vi "goto_mem_pos.vi"(6 "Speed (um/s)":i32, 8 "error in (no error)":errorcluster, 9 "storage_id":i32, 10 "device ID":i32, 11 "Handle in":i64) -> (0 "error out":errorcluster, 2 "Return (<0 is error)":i32, 3 "Handle out":i64)   [LabVIEW 2016, in "OSB_uMp_library.lvlib"]
doc: "Sends uMp to a previously stored position"
uses:
  OSB_uMp_library.lvlib
  ump.dll
panel:
  # "By Stuart Box at OxSyBio Ltd, 2017\n\nThis software is provided WITHOUT ANY WARRANTY; without even the implied warranty of MERCHANTABILITY or FITNESS FOR A PARTICULAR PURPOSE.\n\ninfo@oxsybio.com\n\nOxSyBio Ltd, The Walbrook Building, 25 Walbrook, London, EC4N 8AF"
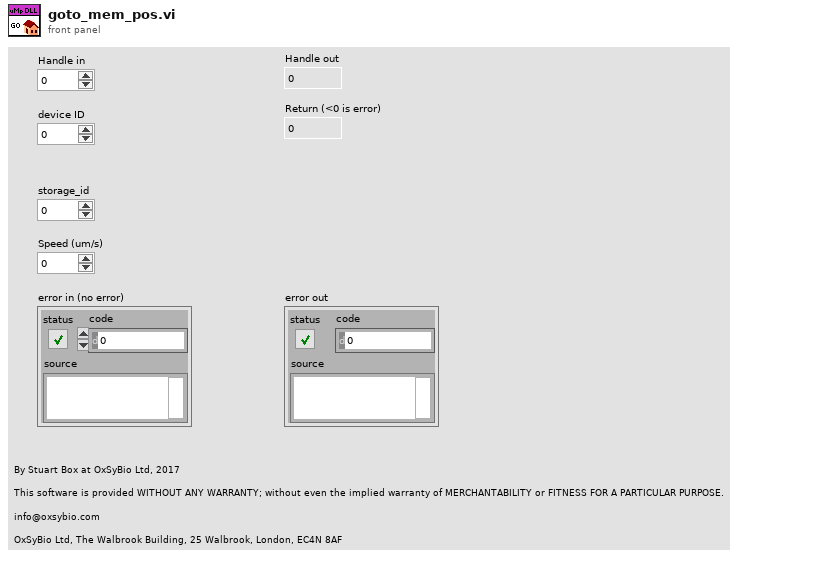
[diagram p1: front panel]
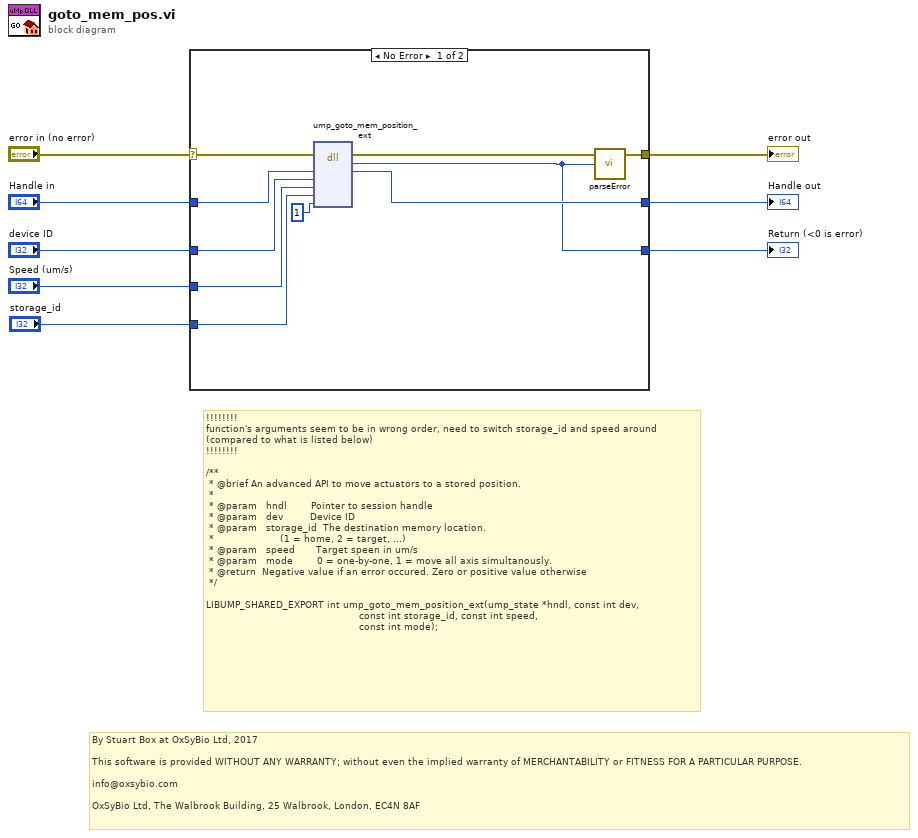
[diagram p0: block diagram]
diagram:
  # "By Stuart Box at OxSyBio Ltd, 2017\n\nThis software is provided WITHOUT ANY WARRANTY; without even the implied warranty of MERCHANTABILITY or FITNESS FOR A PARTICULAR PURPOSE.\n\ninfo@oxsybio.com\n\nOxSyBio Ltd, The Walbrook Building, 25 Walbrook, London, EC4N 8AF"
  # "!!!!!!!!\nfunction's arguments seem to be in wrong order, need to switch storage_id and speed around\n(compared to what is listed below)\n!!!!!!!!\n\n/**\n * @brief An advanced API to move actuators to a stored position.\n *\n * @param   hndl        Pointer to session handle\n * @param   dev         Device ID\n * @param   storage_id  The destination memory location.\n *                      (1 = home, 2 = target, ...)\n * @param   speed       Target speen in um/s\n * @param   mode        0 = one-by-one, 1 = move all axis simultanously.\n * @return  Negative value if an error occured. Zero or positive value otherwise\n */\n\nLIBUMP_SHARED_EXPORT int ump_goto_mem_position_ext(ump_state *hndl, const int dev,\n                                                   const int storage_id, const int speed,\n                                                   const int mode);"
  n1 = case shown="No Error" "error in (no error)" {
    selector: "error in (no error)" -> [w14 w20]
    tunnel: [w9 _] -> w8
    tunnel: [w10 w20] -> w7
    tunnel: "storage_id" -> [w12 _]
    tunnel: "device ID" -> [w18 _]
    tunnel: "Handle in" -> [w17 w19]
    tunnel: "Speed (um/s)" -> [w13 _]
    tunnel: [w15 w19] -> w2
    frame No Error {
      n2 = dll-call lib="C:/Users/Stu/Desktop/OSB LabVIEW uMp/uMp_library/ump.dll" fn="ump_goto_mem_position_ext"(error in=w14, "handle"=w17, "dev"=w18, "speed"=w13, "storage_id"=w12, "mode"=1) -> (error out=w11:errorcluster, "return"=w9:i32, "handle"=w15:i64)  [unwired: 6 in, 1 out]
      n3 = call "parseError.vi"("Error In"=w11, "ump dll return value (<0 is error)"=w9) -> ("Error Out"=w10:errorcluster)  [unwired: 24 in, 1 out]
    }
    frame Error {
    }
  }
  "Return (<0 is error)" <- w8
  "error out" <- w7
  "Handle out" <- w2
